vi "Transparent Image Overlay.vi"() -> ()   [LabVIEW 2012, in "Picture Box Tools.lvlib"]
uses:
  Picture Box Tools.lvlib
  <vilib>/picture/picture.llb/imagedata.ctl
  <vilib>/picture/picture.llb/Draw True-Color Pixmap.vi
panel:
  in  "image data":T1={"image type"=0, "image depth"=24, "image"=array[49050 elements], "mask"=[], "colors"=[], "Rectangle"={"left"=0, "top"=0, "right"=109, "bottom"=150}} caption="图像数据"
  in  "Circle Overlays":T2(array[cluster])=[{"pixel center"={"horizontal"=50, "vertical"=50}, "radius"=30, "circle color"=16711680}, {"pixel center"={"horizontal"=20, "vertical"=20}, "radius"=30, "circle color"=327900}, {"pixel center"={"horizontal"=100, "vertical"=100}, "radius"=30, "circle color"=1985280}]
  in  "Transparency Factor":dbl(slide)=0.5757575757575758 min=0.0 max=1.0 step=0.05 scale=0.0..1.0
  out "Original Image":picture
  out "Overlay":picture
  out "Final Image":picture
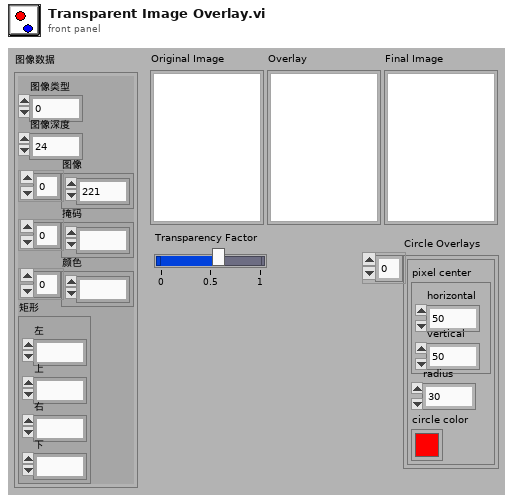
[diagram p1: front panel]
types:
  T1 = typedef "imagedata.ctl" = cluster{"image type":i32, "image depth":i32, "image":u8[], "mask":u8[], "colors":u32[], "Rectangle":cluster{"left":i16, "top":i16, "right":i16, "bottom":i16}}
  T2 = cluster{"pixel center":cluster{"horizontal":i16, "vertical":i16}, "radius":i16, "circle color":u32}[]
  T3 = cluster{"left":i16, "top":i16, "right":i16, "bottom":i16}
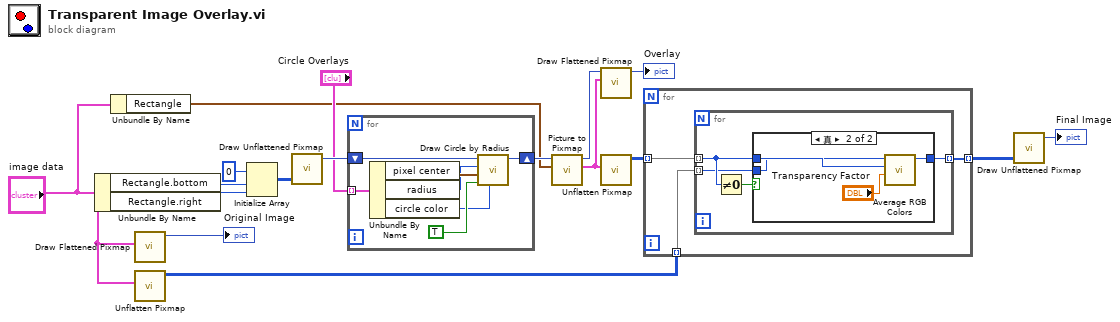
[diagram p0: block diagram]
diagram:
  n1 = Unbundle By Name("image data") -> ("Rectangle.bottom"=w16:i16, "Rectangle.right"=w15:i16)
  n2 = Unbundle By Name("image data") -> ("Rectangle"=w1:T3)
  n3 = call <vilib>:"Draw Flattened Pixmap.vi"("image data"="image data") -> ("new picture"=→"Original Image":picture)  [unwired: 8 in]
  n4 = call <vilib>:"Unflatten Pixmap.vi"("image data"="image data") -> ("24-bit pixmap"=w13:u32[][])  [unwired: 4 in, 6 out]
  n5 = Initialize Array(u32 0, w16, w15) -> (w14:u32[][])
  n6 = call-poly <vilib>:"Draw Unflattened Pixmap.vi"("data (RGB format)"=w14) -> ("new picture"=w8:picture)  [unwired: 8 in]
  n7 = for {
    shift-right: [w22] -> w6
    shift-left: w8 -> [w23]
    tunnel: "Circle Overlays" -> [w21] mode=indexing
    n8 = Unbundle By Name(w21) -> ("pixel center"=w20:cluster{"horizontal":i16, "vertical":i16}, "radius"=w19:i16, "circle color"=w18:u32)
    n9 = call <vilib>:"Draw Circle by Radius.vi"("color(black)"=w18, "fill?(F)"=TRUE, "pixel center"=w20, "radius"=w19, "picture"=w23) -> ("new picture"=w22:picture)  [unwired: 6 in]
  }
  n10 = call <vilib>:"Picture to Pixmap.vi"("rect"=w1, "picture"=w6) -> ("image data"=w9:T1, "new picture"=w4:picture)  [unwired: 8 in]
  n11 = call <vilib>:"Draw Flattened Pixmap.vi"("image data"=w9, "picture"=w4) -> ("new picture"=→"Overlay":picture)  [unwired: 7 in]
  n12 = call <vilib>:"Unflatten Pixmap.vi"("image data"=w9) -> ("24-bit pixmap"=w11:u32[][])  [unwired: 4 in, 6 out]
  n13 = for {
    tunnel: w13 -> [w26] mode=indexing
    tunnel: w11 -> [w27] mode=indexing
    tunnel: [w25] -> w10 mode=indexing
    n14 = for {
      tunnel: w27 -> [w30] mode=indexing
      tunnel: w26 -> [w29] mode=indexing
      tunnel: [w28] -> w25 mode=indexing
      n15 = Not Equal To 0?(x=w30) -> (x != 0?=w31:bool)
      n16 = case shown="真" w31 {
        tunnel: w30 -> [_ w36]
        tunnel: w29 -> [w32 w35]
        tunnel: [w32 w34] -> w28
        frame False {
        }
        frame True {
          n17 = call "Average RGB Colors.vi"("Transparency Factor"="Transparency Factor", "x"=w36, "y"=w35) -> ("result"=w34:u32)  [unwired: 8 in]
        }
      }
    }
  }
  n18 = call-poly <vilib>:"Draw Unflattened Pixmap.vi"("data (RGB format)"=w10) -> ("new picture"=→"Final Image":picture)  [unwired: 8 in]
